vi "sub_DL950_run.vi"(8 "error in":errorcluster) -> (0 "error out":errorcluster)   [LabVIEW 2019]
uses:
  _ctrl/fgv_DL950.ctl
  _ctrl/rw.ctl
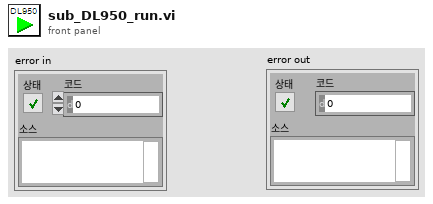
[diagram p1: front panel]
types:
  T1 = typedef "rw.ctl" = enum16{"read", "write"}
  T2 = typedef "fgv_DL950.ctl" = enum16{"init", "config", "Set-NCh", "setapply", "trigger", "read", "time-div", "wave-aquis", "start", "query", "abort", "set_items", "reset_items", "read_items", "percent_rise", "trigger_single", "stop", "close"}
  T3 = typedef "DL950_config.ctl" = cluster{"Timeout":u32, "Time Div":i32, "Acq Mode":i32, "Record Len":i32, "Record Num":i32, "Start Point":i64, "End Poin":i64, "Visa":refnum<visa-resource-name>, "Config Voltage":cluster{"Enable":bool, "Ch":u16, "V Div":i32, "Coupling":i32, "Probe":i32, "Act.Items":bool, "items":i32[]}[], "Trigger on":bool, "Trigger Level":dbl, "Reset":bool, "Config Temp":cluster{"Channel":u16, "Burn Out":bool, " Type ":i32}[], "Trigger Mode":i32, "Trigger Position":dbl, "Trigger Slope":i32, "Trigger Source ":i32, "Start Point (-5.00)":dbl, "End Point (5.00)":dbl}
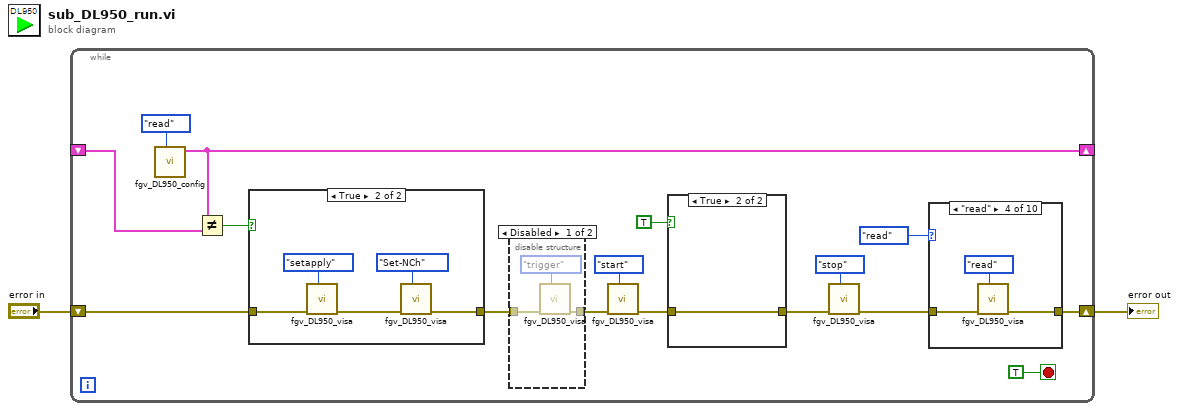
[diagram p0: block diagram]
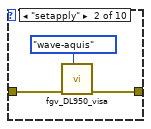
[diagram p6: hidden frame]
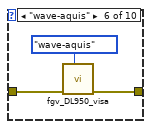
[diagram p9: hidden frame]
diagram:
  n1 = while {
    shift-right: [w15] -> w2
    shift-left: "error in" -> [w11]
    shift-right: [w4] -> _
    shift-left: _ -> [w5]
    stop <- TRUE stop-if-true
    n2 = call "fgv_DL950_config.vi"("cmd"=rw."read") -> ("config 2"=w4:T3)  [unwired: 9 in, 1 out]
    n3 = Not Equal?(x=w4, y=w5) -> (x != y?=w3:bool)
    n4 = case shown="True" w3 {
      tunnel: w11 -> [w25 w30]
      tunnel: [w25 w29] -> w17
      frame False {
      }
      frame True {
        n5 = call "fgv_DL950_visa.vi"("cmd"=fgv_DL950."setapply", "error in"=w30) -> ("error out"=w26:errorcluster)  [unwired: 7 in, 2 out]
        n6 = call "fgv_DL950_visa.vi"("cmd"=fgv_DL950."Set-NCh", "error in"=w26) -> ("error out"=w29:errorcluster)  [unwired: 7 in, 2 out]
      }
    }
    n7 = disable-structure shown="Disabled" {
      disable-tunnel: [w21 w22] -> w18
      disable-tunnel: w17 -> [w20 w22]
      frame Disabled {
        n8 = call "fgv_DL950_visa.vi"("cmd"=fgv_DL950."trigger", "error in"=w20) -> ("error out"=w21:errorcluster)  [unwired: 7 in, 2 out]
      }
      frame Enabled {
      }
    }
    n9 = call "fgv_DL950_visa.vi"("cmd"=fgv_DL950."start", "error in"=w18) -> ("error out"=w13:errorcluster)  [unwired: 7 in, 2 out]
    n10 = case shown="True" TRUE {
      tunnel: w13 -> [w23 w24]
      tunnel: [w23 w24] -> w14
      frame False {
      }
      frame True {
      }
    }
    n11 = call "fgv_DL950_visa.vi"("cmd"=fgv_DL950."stop", "error in"=w14) -> ("error out"=w10:errorcluster)  [unwired: 7 in, 2 out]
    n12 = case shown="\"read\"" fgv_DL950."read" ("cmd") {
      tunnel: [_ w32 _ w35 _ w37 _ _ _ _] -> w15
      tunnel: w10 -> [_ w31 _ w34 _ w38 _ _ _ _]
      frame "init", Default {
      }
      frame "setapply" {
        n13 = call "fgv_DL950_visa.vi"("cmd"=fgv_DL950."wave-aquis", "error in"=w31) -> ("error out"=w32:errorcluster)  [unwired: 7 in, 2 out]
      }
      frame "config" {
      }
      frame "read" {
        n14 = call "fgv_DL950_visa.vi"("cmd"=fgv_DL950."read", "error in"=w34) -> ("error out"=w35:errorcluster)  [unwired: 7 in, 2 out]
      }
      frame "time-div" {
      }
      frame "wave-aquis" {
        n15 = call "fgv_DL950_visa.vi"("cmd"=fgv_DL950."wave-aquis", "error in"=w38) -> ("error out"=w37:errorcluster)  [unwired: 7 in, 2 out]
      }
      frame "start" {
      }
      frame "abort" {
      }
      frame "stop" {
      }
      frame "close" {
      }
    }
  }
  "error out" <- w2
